vi "JSON Tree to Init State.vi"(8 "error in (no error)":errorcluster, 11 "JSON Tree Out Passthrough":variant) -> (0 "error out":errorcluster, 2 "Initial State":T1, 3 "JSON Tree Out":variant)   [LabVIEW 2015, in "SLSC Switch.lvlib" / "SLSC Switch.lvclass"]
uses:
  SLSC Switch.lvclass
  Controls/JSON.InitialState.ctl
  <vilib>/LVH/i3 JSON/JSON Parsing/Get Object Parameter Files/Get Object Parameter - Object.vi
  <vilib>/LVH/i3 JSON/i3-json.lvlib
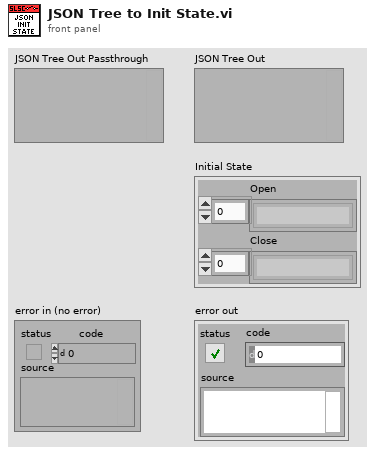
[diagram p1: front panel]
types:
  T1 = typedef "SLSC Switch.lvlib/SLSC Switch.lvclass/JSON.InitialState.ctl" = cluster{"Open":string[], "Close":string[]}
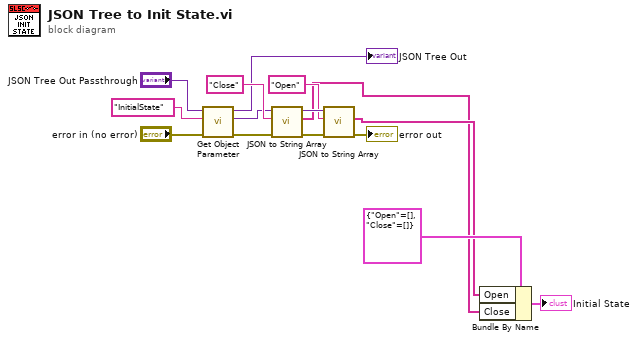
[diagram p0: block diagram]
diagram:
  n1 = call-poly <vilib>:"Get Object Parameter.vi"("error in (no error)"="error in (no error)", "Parameter Name"="InitialState", "JSON Tree In (JSON Object)"="JSON Tree Out Passthrough") -> ("error out"=w14:errorcluster, "JSON Object"=w11:variant, "JSON Tree Out Passthrough"=→"JSON Tree Out":variant)  [unwired: 5 in, 1 out]
  n2 = call "JSON to String Array.vi"("error in (no error)"=w14, "Parameter Name"="Close", "JSON Tree In"=w11) -> ("error out"=w15:errorcluster, "Array"=w2:string[], "JSON Tree Out"=w12:variant)  [unwired: 6 in]
  n3 = call "JSON to String Array.vi"("error in (no error)"=w15, "Parameter Name"="Open", "JSON Tree In"=w12) -> ("error out"=→"error out":errorcluster, "Array"=w3:string[])  [unwired: 6 in, 1 out]
  n4 = Bundle By Name(cluster=T1 {"Open"=[], "Close"=[]} ("InitialState"), "Open"=w3, "Close"=w2) -> (→"Initial State":T1)
